vi "Initialize Memory Blocks.vi"() -> (0 "Memory":T1)   [LabVIEW 2017]
uses:
  Memory Block Channels.ctl
  MemoryBlocks.ctl
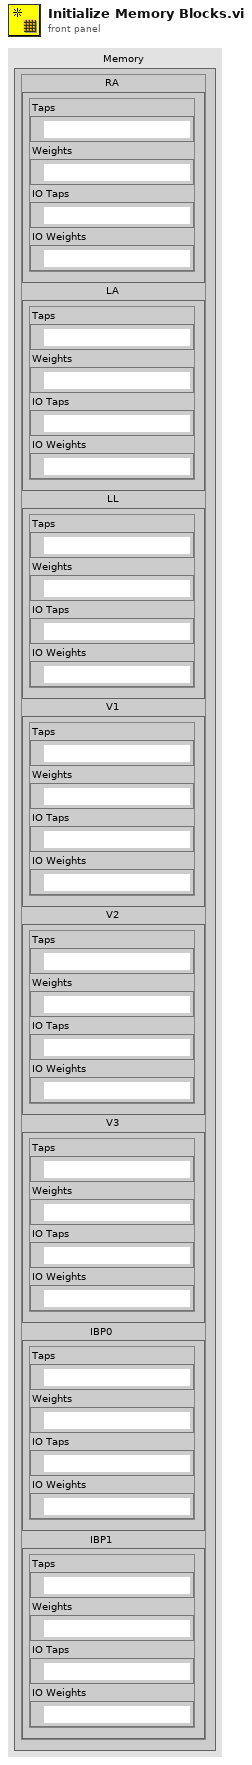
[diagram p1: front panel]
types:
  T1 = typedef "Memory Block Channels.ctl" = cluster{"RA":T2, "LA":T2, "LL":T2, "V1":T2, "V2":T2, "V3":T2, "IBP0":T2, "IBP1":T2}
  T2 = typedef "MemoryBlocks.ctl" = cluster{"Taps":refnum<k21>, "Weights":refnum<k21>, "IO Weights":refnum<k21>, "IO Taps":refnum<k21>}
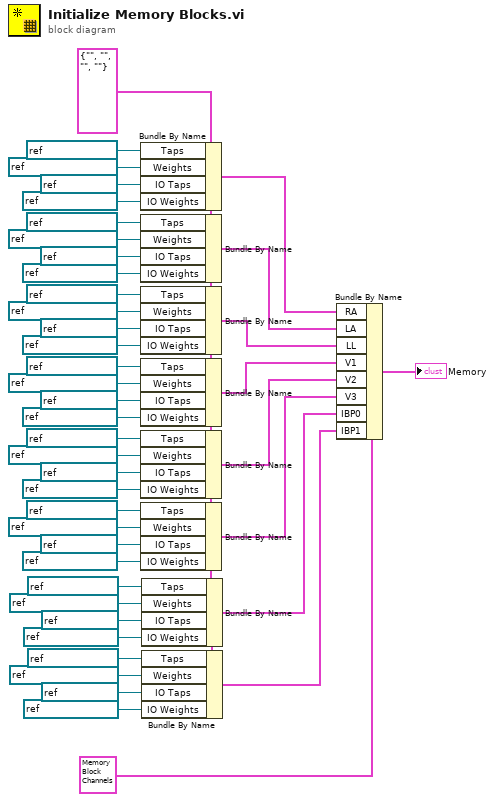
[diagram p0: block diagram]
diagram:
  w5 = T2 {"Taps"="", "Weights"="", "IO Weights"="", "IO Taps"=""} ("output cluster")
  n1 = Bundle By Name(cluster=w5, "Taps"=refnum<k21> "Filter Taps 0" ("Memory"), "Weights"=refnum<k21> "Filter Weights 0" ("Memory In"), "IO Taps"=refnum<k21> "IO Taps 0" ("Memory"), "IO Weights"=refnum<k21> "IO Weights 0" ("Memory In")) -> (w18:T2)
  n2 = Bundle By Name(cluster=w5, "Taps"=refnum<k21> "Filter Taps 1" ("Memory"), "Weights"=refnum<k21> "Filter Weights 1" ("Memory In"), "IO Taps"=refnum<k21> "IO Taps 1" ("Memory"), "IO Weights"=refnum<k21> "IO Weights 1" ("Memory In")) -> (w17:T2)
  n3 = Bundle By Name(cluster=w5, "Taps"=refnum<k21> "Filter Taps 2" ("Memory"), "Weights"=refnum<k21> "Filter Weights 2" ("Memory In"), "IO Taps"=refnum<k21> "IO Taps 2" ("Memory"), "IO Weights"=refnum<k21> "IO Weights 2" ("Memory In")) -> (w16:T2)
  n4 = Bundle By Name(cluster=w5, "Taps"=refnum<k21> "Filter Taps 3" ("Memory"), "Weights"=refnum<k21> "Filter Weights 3" ("Memory In"), "IO Taps"=refnum<k21> "IO Taps 3" ("Memory"), "IO Weights"=refnum<k21> "IO Weights 3" ("Memory In")) -> (w15:T2)
  n5 = Bundle By Name(cluster=w5, "Taps"=refnum<k21> "Filter Taps 4" ("Memory"), "Weights"=refnum<k21> "Filter Weights 4" ("Memory In"), "IO Taps"=refnum<k21> "IO Taps 4" ("Memory"), "IO Weights"=refnum<k21> "IO Weights 4" ("Memory In")) -> (w14:T2)
  n6 = Bundle By Name(cluster=w5, "Taps"=refnum<k21> "Filter Taps 5" ("Memory"), "Weights"=refnum<k21> "Filter Weights 5" ("Memory In"), "IO Taps"=refnum<k21> "IO Taps 5" ("Memory"), "IO Weights"=refnum<k21> "IO Weights 5" ("Memory In")) -> (w13:T2)
  n7 = Bundle By Name(cluster=w5, "Taps"=refnum<k21> "Filter Taps 6" ("Memory"), "Weights"=refnum<k21> "Filter Weights 6" ("Memory In"), "IO Taps"=refnum<k21> "IO Taps 6" ("Memory"), "IO Weights"=refnum<k21> "IO Weights 6" ("Memory In")) -> (w2:T2)
  n8 = Bundle By Name(cluster=w5, "Taps"=refnum<k21> "Filter Taps 7" ("Memory"), "Weights"=refnum<k21> "Filter Weights 7" ("Memory In"), "IO Taps"=refnum<k21> "IO Taps 7" ("Memory"), "IO Weights"=refnum<k21> "IO Weights 7" ("Memory In")) -> (w1:T2)
  n9 = Bundle By Name(cluster=T1 {"RA"={"Taps"="", "Weights"="", "IO Weights"="", "IO Taps"=""}, "LA"={"Taps"="", "Weights"="", "IO Weights"="", "IO Taps"=""}, "LL"={"Taps"="", "Weights"="", "IO Weights"="", "IO Taps"=""}, "V1"={"Taps"="", "Weights"="", "IO Weights"="", "IO Taps"=""}, "V2"={"Taps"="", "Weights"="", "IO Weights"="", "IO Taps"=""}, "V3"={"Taps"="", "Weights"="", "IO Weights"="", "IO Taps"=""}, "IBP0"={"Taps"="", "Weights"="", "IO Weights"="", "IO Taps"=""}, "IBP1"={"Taps"="", "Weights"="", "IO Weights"="", "IO Taps"=""}} ("output cluster"), "RA"=w18, "LA"=w17, "LL"=w16, "V1"=w15, "V2"=w14, "V3"=w13, "IBP0"=w2, "IBP1"=w1) -> (→"Memory":T1)
